vi "PicoScope4000RunBlock.vi"(5 "Oversample":i16, 7 "Acquisition Settings":T1 {"postTriggerSamples" format="%_6p"; "preTriggerSamples" format="%_6p"}, 8 "error in (no error)":errorcluster, 11 "handle in":i16) -> (0 "error out":errorcluster, 3 "handle out":i16, 4 "timeIndisposedMs":dbl, 6 "Total Requested Samples":u64)   [LabVIEW 2009]
doc: "Calls RunBlock"
uses:
  ps4000.dll
  shared/Acquisition Settings.ctl
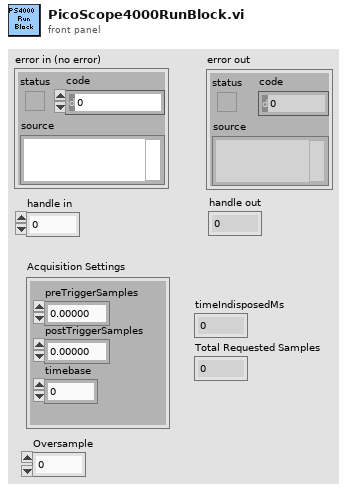
[diagram p1: front panel]
types:
  T1 = typedef "Acquisition Settings.ctl" = cluster{"preTriggerSamples":u64, "postTriggerSamples":u64, "timebase":u32}
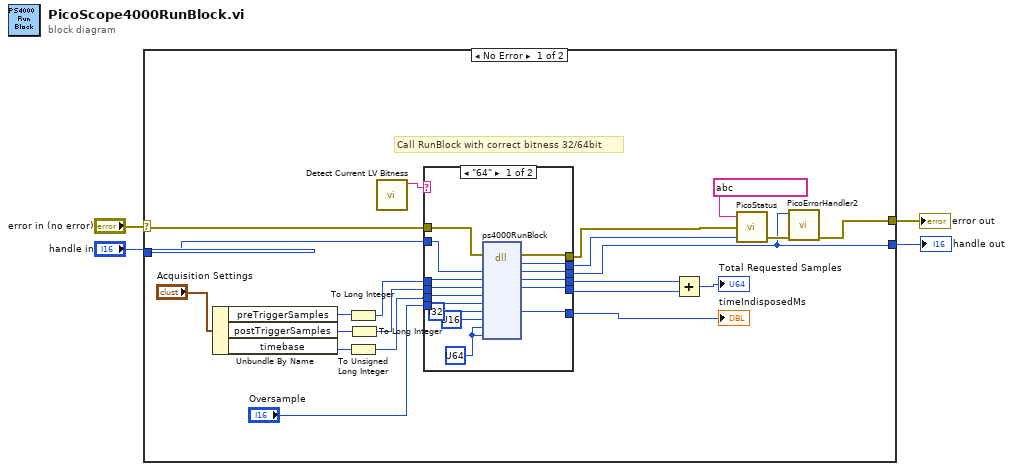
[diagram p0: block diagram]
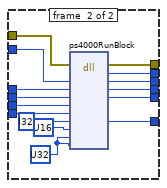
[diagram p2: hidden frame]
diagram:
  n1 = case shown="No Error" "error in (no error)" {
    selector: "error in (no error)" -> [w16 w57]
    tunnel: [w22 w57] -> w2
    tunnel: "handle in" -> [w15 w56]
    tunnel: [w9 w56] -> w3
    frame #0 {
      # "Call RunBlock with correct bitness 32/64bit"
      n2 = Unbundle By Name("Acquisition Settings") -> ("preTriggerSamples"=w20:u64, "postTriggerSamples"=w18:u64, "timebase"=w19:u32)
      n3 = To Long Integer(number=w20) -> (32bit integer=w14:i32)
      n4 = To Unsigned Long Integer(number=w19) -> (unsigned 32bit integer=w12:u32)
      n5 = To Long Integer(number=w18) -> (32bit integer=w13:i32)
      n6 = call "Detect Current LV Bitness.vi"() -> ("bitness"=w17:string)  [unwired: 11 in]
      n7 = case shown="\"64\"" w17 {
        tunnel: [w29 w55] -> w9
        tunnel: [w28 w54] -> w8
        tunnel: [w27 w53] -> w7
        tunnel: w12 -> [w36 w52]
        tunnel: w14 -> [w38 w51]
        tunnel: w13 -> [w37 w50]
        tunnel: [w30 w49] -> w10
        tunnel: [w31 w48] -> w11
        tunnel: w16 -> [w40 w43]
        tunnel: w15 -> [w39 w42]
        tunnel: "Oversample" -> [w35 w47]
        tunnel: [w26 w41] -> w6
        frame #0 {
          w32 = u64 ? ("lpReady")
          n8 = dll-call lib="ps4000.dll" fn="ps4000RunBlock" ("ps3000.dll:_ps3000_open_unit@0")(error in=w40, "handle"=w39, "preTriggerSamples"=w38, "postTriggerSamples"=w37, "timebase"=w36, "oversample"=w35, "timeindisposed"=i32 ?, "segmentIndex"=u16 ?, "lpReady"=w32, "pParameter"=w32) -> (error out=w31:errorcluster, "PICO_STATUS"=w30:u32, "handle"=w29:i16, "preTriggerSamples"=w28:i32, "postTriggerSamples"=w27:i32, "timeindisposed"=w26:i32)  [unwired: 7 in, 1 out]
        }
        frame #1 {
          w44 = u32 ? ("lpReady")
          n9 = dll-call lib="ps4000.dll" fn="ps4000RunBlock" ("ps3000.dll:_ps3000_open_unit@0")(error in=w43, "handle"=w42, "preTriggerSamples"=w51, "postTriggerSamples"=w50, "timebase"=w52, "oversample"=w47, "timeindisposed"=i32 ?, "segmentIndex"=u16 ?, "lpReady"=w44, "pParameter"=w44) -> (error out=w48:errorcluster, "PICO_STATUS"=w49:u32, "handle"=w55:i16, "preTriggerSamples"=w54:i32, "postTriggerSamples"=w53:i32, "timeindisposed"=w41:i32)  [unwired: 7 in, 1 out]
        }
      }
      "timeIndisposedMs" <- w6
      n10 = Add(x=w8, y=w7) -> (x+y=→"Total Requested Samples":i32)
      n11 = call "PicoStatus.vi"("PICO STATUS"=w10, "error in"=w11, "source"=string ?) -> ("error out"=w23:errorcluster)
      n12 = call "PicoErrorHandler2.vi"("error in (no error)"=w23, "handle In"=w9) -> ("error out"=w22:errorcluster)  [unwired: 9 in]
    }
    frame #1 {
    }
  }
  "error out" <- w2
  "handle out" <- w3
